vi "Load App.vi"   [LabVIEW 2020]
doc: "Load the application into memory and start it running. The input notifier is used to send text to the splash screen to tell the user what stage the load process is in."
uses:
  State Pattern UI/State Pattern UI/State Pattern UI.lvclass
  C:/Program Files (x86)/National Instruments/LabVIEW 2020/vi.lib/ActorFramework/Actor/Actor.lvclass
  <vilib>/ActorFramework/Message Queue/Message Queue.lvclass/Message Queue.ctl
  <vilib>/ActorFramework/Actor/Actor.lvclass
  <vilib>/ActorFramework/Message Queue/Message Queue.lvclass
panel:
  # "Overview:  Demonstrates a State Pattern Actor.\nRequirements:  LabVIEW Full Development System, Actor Framework 4.1\nInstructions:  Run the VI."
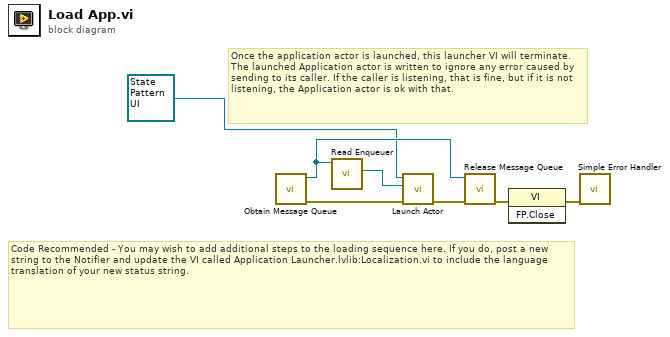
[diagram p0: block diagram]
diagram:
  # "Once the application actor is launched, this launcher VI will terminate. The launched Application actor is written to ignore any error caused by sending to its caller. If the caller is listening, that is fine, but if it is not listening, the Application actor is ok with that."
  # "Code Recommended - You may wish to add additional steps to the loading sequence here. If you do, post a new string to the Notifier and update the VI called Application Launcher.lvlib:Localization.vi to include the language translation of your new status string."
  n1 = call <vilib>:"Obtain Message Queue.vi"() -> ("error out"=w5:errorcluster, "Message Queue"=w4:refnum<class "Message Queue.lvclass">)  [unwired: 10 in]
  n2 = call <vilib>:"Read Enqueuer.vi"("Message Queue"=w4) -> ("Message Enqueuer"=w7:refnum<class "Message Enqueuer.lvclass">)  [unwired: 10 in]
  n3 = call <vilib>:"Launch Actor.vi"("error in (no error)"=w5, "Actor-to-Caller Enqueuer"=w7, "Actor"=refnum<class "State Pattern UI.lvclass"> refnum ("My Application.lvclass")) -> ("error out"=w6:errorcluster)  [unwired: 7 in, 1 out]
  n4 = call <vilib>:"Release Message Queue.vi"("error in (no error)"=w6, "Message Queue"=w4) -> ("error out"=w2:errorcluster)  [unwired: 8 in, 1 out]
  n5 = invoke class="VI" method="FP.Close"(error in=w2) -> (error out=w1:errorcluster)  [unwired: 2 in, 2 out]
  n6 = call <vilib>:"Simple Error Handler.vi"("error in (no error)"=w1) -> ()  [unwired: 4 in, 5 out]
